vi "User_Defined_Test_NewTarget.vi"() -> (3 "Unit Test Framework Results":T1)   [LabVIEW 2016]
doc: "Use this template to create a user-defined test VI. Define your test requirements and wire the results to the <b>Result (Test)</b> control. Do not modify the <b>Unit Test Framework Results</b> indicator."
uses:
  <vilib>/utf/common/utf_test_result_troll.ctl
  <vilib>/utf/common/utf_test_result.ctl
  <vilib>/utf/common/utf_test_result_failure.ctl
  <vilib>/utf/common/utf_test_comparison_operators.ctl
  <vilib>/utf/common/utf_vi_tag.ctl
  <vilib>/Control Software Solutions Ltd/UTF Helper/SubVIs/UTF Boolean Equals.vi
  MyPAM Controller/controllerLibrary.lvlib
  <vilib>/Control Software Solutions Ltd/UTF Helper/Unit Test Helper.lvlib
  <vilib>/utf/NI_UnitTestFramework.lvlib
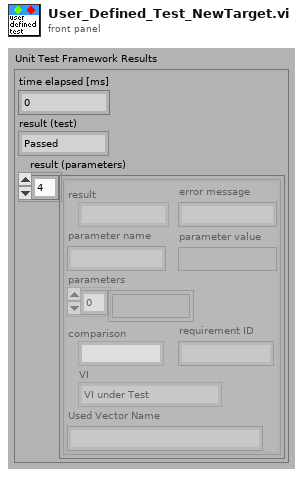
[diagram p1: front panel]
types:
  T1 = typedef "NI_UnitTestFramework.lvlib/utf_test_result_troll.ctl" = cluster{"time elapsed [ms]":u32, "result (test)":T2, "result (parameters)":T3[]}
  T2 = typedef "NI_UnitTestFramework.lvlib/utf_test_result.ctl" = enum16{"Passed", "Failed", "Error", "Skipped", "Not Processed"}
  T3 = typedef "NI_UnitTestFramework.lvlib/utf_test_result_failure.ctl" = cluster{"result":T2, "error message":string, "parameter name":string, "parameter value":variant, "parameters":variant[], "comparison":T4, "requirement ID":string, "VI":T5, "Used Vector Name":string}
  T4 = typedef "NI_UnitTestFramework.lvlib/utf_test_comparison_operators.ctl" = enum16{"=", "!=", ">", ">=", "<", "<=", "range", "symmetric tolerance", "asymmetric tolerance", "string contains", "string not contain", "array size", "string length", "array range", "by element", "array range (limit array)", "user-defined", "array contains", "array not contain", "vector length", "= (elm)", "!= (elm)", "= (case insensitive)", "!= (case insensitive)"}
  T5 = typedef "NI_UnitTestFramework.lvlib/utf_vi_tag.ctl" = enum16{"Setup VI", "VI under Test", "Teardown VI"}
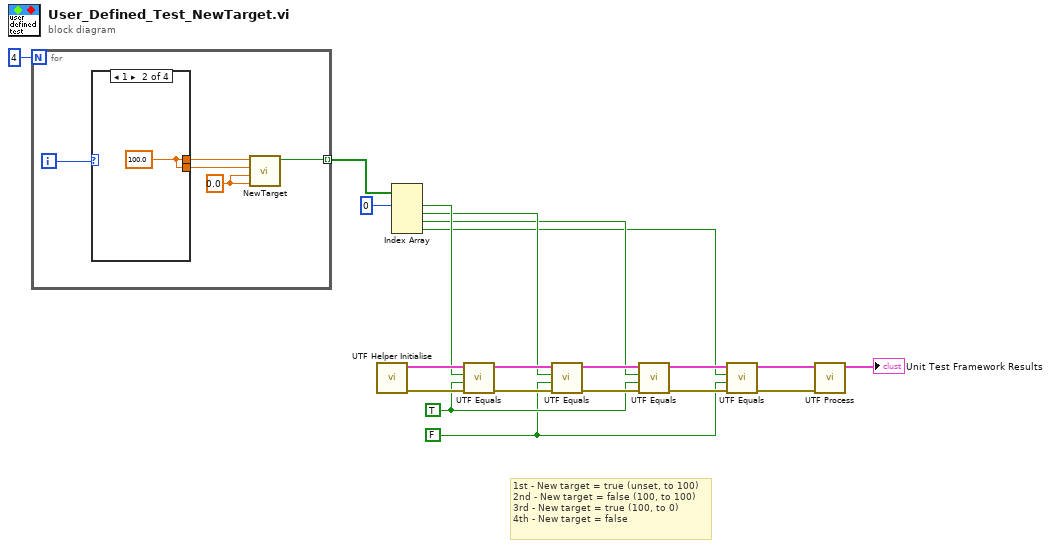
[diagram p0: block diagram]
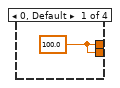
[diagram p2: hidden frame]
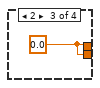
[diagram p3: hidden frame]
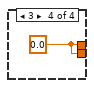
[diagram p4: hidden frame]
diagram:
  w1 = FALSE
  w2 = TRUE
  # "1st - New target = true (unset, to 100)\n2nd - New target = false (100, to 100)\n3rd - New target = true (100, to 0)\n4th - New target = false"
  n1 = for {
    N: 4 -> [_]
    tunnel: [w24] -> w8 mode=indexing
    i -> [w25]
    w23 = 0.0
    n2 = case shown="1" w25 {
      tunnel: [w26 w27 w28 w29] -> w22
      tunnel: [w26 w27 w28 w29] -> w21
      frame 0, Default {
        w26 = 100.0
      }
      frame 1 {
        w27 = 100.0
      }
      frame 2 {
        w28 = 0.0
      }
      frame 3 {
        w29 = 0.0
      }
    }
    n3 = call "NewTarget.vi"("Current y"=w23, "Current x"=w23, "Target y"=w21, "Target x"=w22) -> ("new target?"=w24:bool)  [unwired: 7 in]
  }
  n4 = call <vilib>:"UTF Helper Initialise.vi"() -> ("error out"=w18:errorcluster, "results array"=w9:T3[])  [unwired: 10 in]
  n5 = Index Array(array=w8, index #1=0 ("index")) -> (element #1=w7:bool, element #2=w5:bool, element #3=w4:bool, element #4=w3:bool)  [unwired: 3 in]
  n6 = call-poly <vilib>:"UTF Equals.vi"("error in (no error)"=w18, "Test Value"=w2, "Input"=w7, "Input Results"=w9) -> ("error out"=w17:errorcluster, "Output Results"=w10:T3[])  [unwired: 6 in]
  n7 = call-poly <vilib>:"UTF Equals.vi"("error in (no error)"=w17, "Test Value"=w1, "Input"=w5, "Input Results"=w10) -> ("error out"=w16:errorcluster, "Output Results"=w11:T3[])  [unwired: 6 in]
  n8 = call-poly <vilib>:"UTF Equals.vi"("error in (no error)"=w16, "Test Value"=w2, "Input"=w4, "Input Results"=w11) -> ("error out"=w15:errorcluster, "Output Results"=w12:T3[])  [unwired: 6 in]
  n9 = call-poly <vilib>:"UTF Equals.vi"("error in (no error)"=w15, "Test Value"=w1, "Input"=w3, "Input Results"=w12) -> ("error out"=w14:errorcluster, "Output Results"=w13:T3[])  [unwired: 6 in]
  n10 = call <vilib>:"UTF Process.vi"("error in (no error)"=w14, "results array"=w13) -> ("Unit Test Framework Results"=→"Unit Test Framework Results":T1)  [unwired: 9 in]
